vi "run.vi"(8 "error in (no error)":errorcluster, 11 "DL090503StimulatorScaffold in":refnum<class "StimulatorDL090503Scaffold.lvclass">) -> (0 "error out":errorcluster, 3 "DL090503StimulatorScaffold out":refnum<class "StimulatorDL090503Scaffold.lvclass">)   [LabVIEW 2010, in "StimulatorDL090503Scaffold.lvclass"]
uses:
  StimulatorDL090503Scaffold.lvclass
  schedule_entry_cluster.ctl
  common/classes/GenericToplevelComponent/GenericToplevelComponent/common_trigger_enum.ctl
  internal_trigger_enum.ctl
  StimulatorDL090503Scaffold.lvclass/StimulatorDL090503Scaffold.ctl
  GenericStimulator/GenericStimulator/GenericStimulator.lvclass
  common/classes/GenericComponent/GenericComponent/class_data.vi
  common/classes/GenericToplevelComponent/GenericToplevelComponent/GenericToplevelComponent.lvclass
  common/classes/GenericComponent/GenericComponent/GenericComponent.lvclass
panel:
  out "last statechart trigger":T1
  out "event loop time-out":i32
  in  "scheduled triggers":T2[](array[typedef])
  out "trigger schedule loop counter":i32
  out "statemachine  error":errorcluster
  out "statechart loop counter":i32
  out "finished?":bool
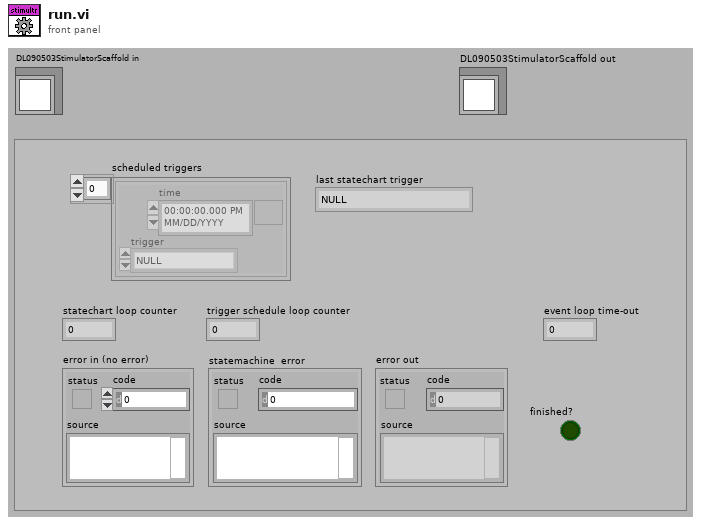
[diagram p1: front panel]
types:
  T1 = typedef "StimulatorDL090503Scaffold.lvclass/internal_trigger_enum.ctl" = enum16{"NULL", "initialise", "terminate", "start sweep", "stop sweep", "start stimulation", "stop stimulation"}
  T2 = typedef "StimulatorDL090503Scaffold.lvclass/schedule_entry_cluster.ctl" = cluster{"time":timestamp, "trigger":T3}
  T3 = typedef "GenericToplevelComponent.lvclass/common_trigger_enum.ctl" = enum16{"NULL", "initialise", "terminate", "fetch command", "fetch data", "attach observer", "register as observer", "detach observer", "acknowledge", "start", "stop", "sweep started", "sweep finished", "experiment started", "experiment stopped"}
  T4 = typedef "main_trigger_enum.ctl" = enum16{"NULL", "initialise", "terminate", "start", "stop", "change objective", "change experimentController", "change imagingMode", "save notebook", "started saving", "finished saving", "expCtr ready", "expCtr missing", "imgMd ready", "imgMd missing", "scanHd ready", "scanHd missing", "DAQ ready", "DAQ missing", "imgAsm ready", "imgAsm missing", "dataColl ready", "dataColl missing", "display ready", "display missing", "analysr ready", "analysr missing", "instrmnt ready", "instrmnt missing", "stimltr ready", "stimltr missing", "stage ready", "stage missing"}
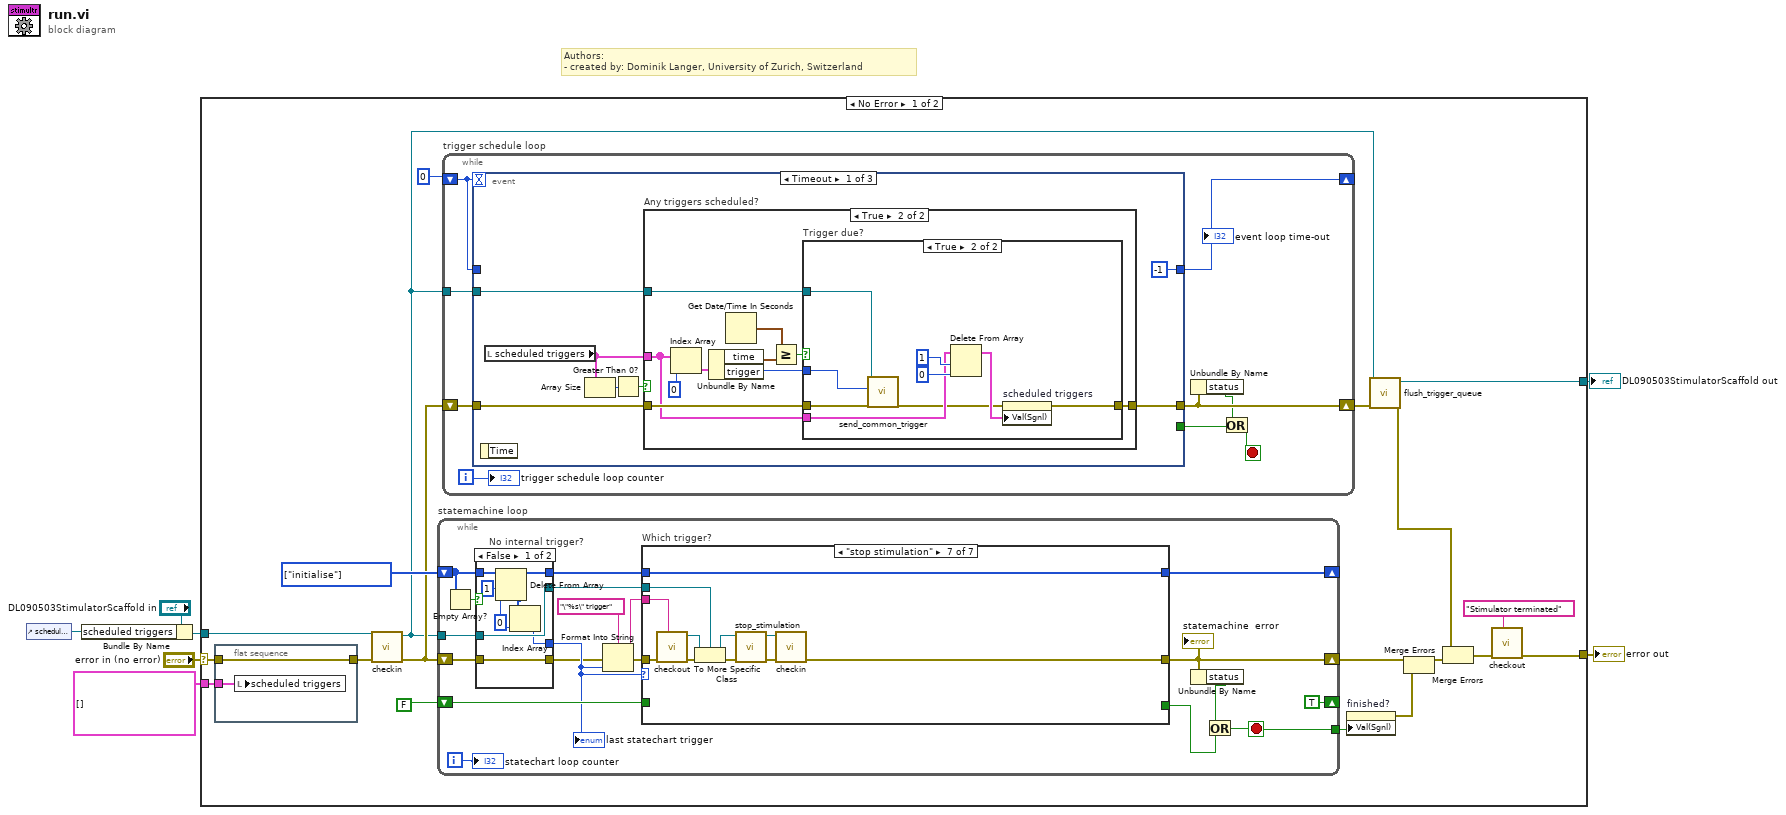
[diagram p0: block diagram]
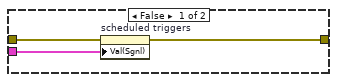
[diagram p3: hidden frame]
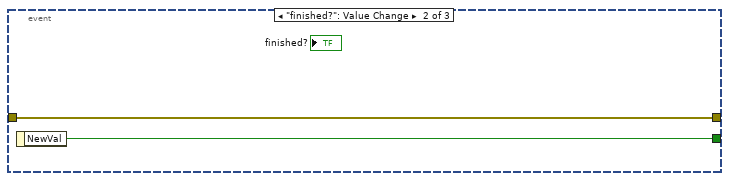
[diagram p4: hidden frame]
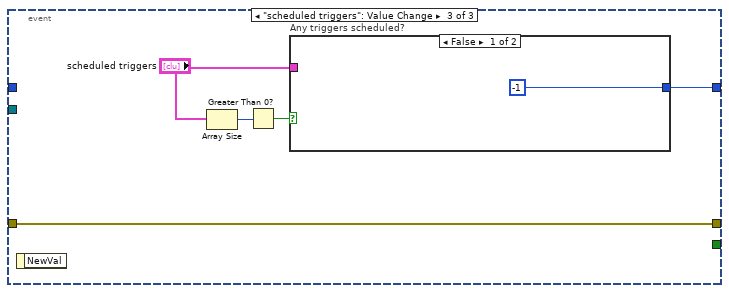
[diagram p5: hidden frame]
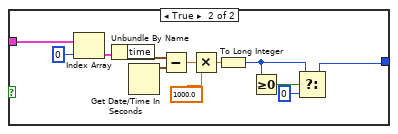
[diagram p6: hidden frame]
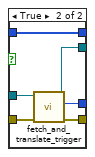
[diagram p7: hidden frame]
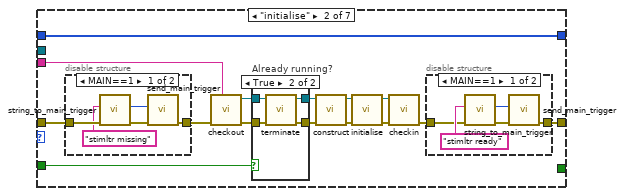
[diagram p9: hidden frame]
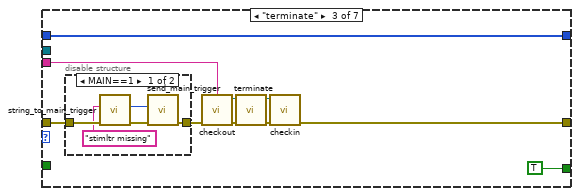
[diagram p13: hidden frame]
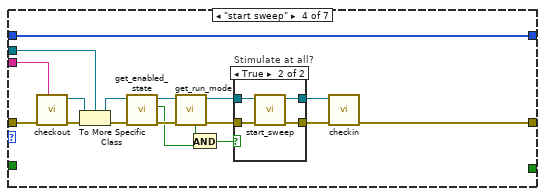
[diagram p15: hidden frame]
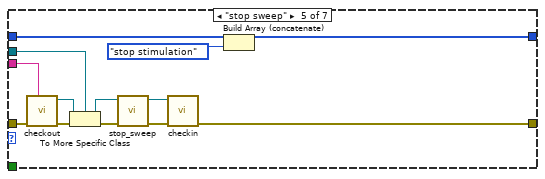
[diagram p17: hidden frame]
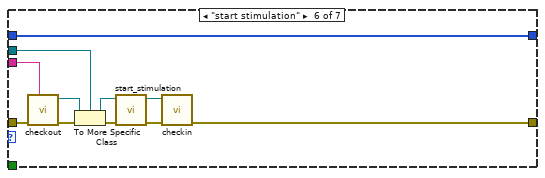
[diagram p18: hidden frame]
diagram:
  # "Authors: \n- created by: Dominik Langer, University of Zurich, Switzerland"
  n1 = control-ref of="scheduled triggers"() -> (w1:refnum<vi>)
  n2 = Bundle By Name(cluster="DL090503StimulatorScaffold in", "scheduled triggers"=w1) -> (w3:refnum<class "StimulatorDL090503Scaffold.lvclass">)
  n3 = case shown="No Error" "error in (no error)" {
    selector: "error in (no error)" -> [w23 w232]
    tunnel: [w15 w232] -> w6
    tunnel: w3 -> [w18 w231]
    tunnel: [w20 w231] -> w5
    tunnel: T2[] [] ("scheduled triggers") -> [w24 _]
    frame No Error {
      w10 = T1[] [enum."initialise"] items=["NULL", "initialise", "terminate", "start sweep", "stop sweep", "start stimulation", "stop stimulation"]
      n4 = flat-sequence {
        tunnel: w24 -> [w28]
        tunnel: w23 -> [w27]
        tunnel: [w27] -> w19
        frame #0 {
          n5 = local write "scheduled triggers"(w28) -> ()
        }
      }
      n6 = call-dynamic "checkin.vi"("error in (no error)"=w19, "GenericStimulator in"=w18) -> ("error out"=w9:errorcluster, "GenericStimulator out"=w8:refnum<class "StimulatorDL090503Scaffold.lvclass">)  [unwired: 8 in]
      n7 = while "statemachine loop" {
        shift-right: [TRUE] -> _
        shift-left: FALSE -> [w101]
        shift-right: [w100] -> w13
        shift-left: w9 -> [w104]
        tunnel: w8 -> [w103]
        tunnel: [w102] -> w17
        shift-right: [w91] -> _
        shift-left: w10 -> [w90]
        i -> [w105]
        stop <- w102 stop-if-true
        n8 = Empty Array?(array=w90) -> (empty?=w89:bool)
        n9 = case "No internal trigger?" shown="False" w89 {
          tunnel: w104 -> [w114 w120]
          tunnel: w103 -> [w113 w119]
          tunnel: [w109 w118] -> w97
          tunnel: [w114 w117] -> w96
          tunnel: [w113 w116] -> w92
          tunnel: w90 -> [w112 w115]
          tunnel: [w111 w115] -> w88
          frame False {
            w108 = 0 ("index")
            n10 = Delete From Array(array=w112, length=1, index=w108) -> (deleted portion=w110:T1[], array with subset deleted=w111:T1[])
            n11 = Index Array(array=w110, index=w108) -> (element=w109:T1)
          }
          frame True {
            n12 = call-dynamic "fetch_and_translate_trigger.vi"("error in (no error)"=w120, "StimulatorDL090503Scaffold in"=w119) -> ("error out"=w117:errorcluster, "statechart trigger"=w118:T1, "StimulatorDL090503Scaffold out"=w116:refnum<class "StimulatorDL090503Scaffold.lvclass">)  [unwired: 6 in, 1 out]
          }
        }
        "last statechart trigger" <- w97
        n13 = Format Into String(format string="\"%s\" trigger", error in=w96, w97) -> (resulting string=w93:string, error out=w95:errorcluster)  [unwired: 1 in]
        n14 = case "Which trigger?" shown="\"stop stimulation\"" w97 {
          tunnel: w95 -> [w122 w125 w157 w184 w200 w210 w223]
          tunnel: w101 -> [_ w128 _ _ _ _ _]
          tunnel: [w122 w126 w159 w183 w199 w209 w220] -> w100
          tunnel: [_ _ TRUE _ _ _ _] -> w99
          tunnel: w93 -> [_ w129 w160 w185 w202 w211 w221]
          tunnel: w92 -> [_ _ _ w182 w201 w212 w222]
          tunnel: w88 -> [w121 w123 w158 w181 w197 w219 w230]
          tunnel: [w121 w123 w158 w181 w196 w219 w230] -> w91
          frame "NULL", Default {
          }
          frame "initialise" {
            n15 = disable-structure shown="MAIN==1" {
              disable-tunnel: w125 -> [w141 w143]
              disable-tunnel: [w142 w143] -> w124
              frame condition #0 (active) {
                n16 = call "string_to_main_trigger.vi"("error in (no error)"=w141, "trigger string"="stimltr missing") -> ("error out"=w140:errorcluster, "main trigger"=w139:T4)  [unwired: 8 in]
                n17 = call "send_main_trigger.vi"("error in (no error)"=w140, "trigger"=w139) -> ("error out"=w142:errorcluster)  [unwired: 9 in]
              }
              frame condition #1 {
              }
            }
            n18 = call "checkout.vi"("locked by?"=w129, "error in (no error)"=w124) -> ("error out"=w134:errorcluster, "GenericStimulator out"=w136:refnum<class "GenericStimulator.lvclass">)  [unwired: 8 out]
            n19 = case "Already running?" shown="True" w128 {
              tunnel: w134 -> [w151 w155]
              tunnel: [w151 w154] -> w135
              tunnel: w136 -> [w150 w153]
              tunnel: [w150 w152] -> w137
              frame False {
              }
              frame True {
                n20 = call-dynamic "terminate.vi"("error in (no error)"=w155, "GenericPlugin in"=w153) -> ("error out"=w154:errorcluster, "GenericPlugin out"=w152:refnum<class "GenericStimulator.lvclass">)  [unwired: 8 out]
              }
            }
            n21 = call-dynamic "construct.vi"("error in (no error)"=w135, "GenericPlugin in"=w137) -> ("error out"=w132:errorcluster, "GenericPlugin out"=w133:refnum<class "GenericStimulator.lvclass">)  [unwired: 2 in, 6 out]
            n22 = call-dynamic "initialise.vi"("error in (no error)"=w132, "GenericPlugin in"=w133) -> ("error out"=w131:errorcluster, "GenericPlugin out"=w130:refnum<class "GenericStimulator.lvclass">)  [unwired: 8 out]
            n23 = call-dynamic "checkin.vi"("error in (no error)"=w131, "GenericStimulator in"=w130) -> ("error out"=w127:errorcluster)  [unwired: 8 in, 1 out]
            n24 = disable-structure shown="MAIN==1" {
              disable-tunnel: w127 -> [w145 w149]
              disable-tunnel: [w148 w149] -> w126
              frame condition #0 (active) {
                n25 = call "string_to_main_trigger.vi"("error in (no error)"=w145, "trigger string"="stimltr ready") -> ("error out"=w144:errorcluster, "main trigger"=w147:T4)  [unwired: 8 in]
                n26 = call "send_main_trigger.vi"("error in (no error)"=w144, "trigger"=w147) -> ("error out"=w148:errorcluster)  [unwired: 9 in]
              }
              frame condition #1 {
              }
            }
          }
          frame "terminate" {
            n27 = disable-structure shown="MAIN==1" {
              disable-tunnel: w157 -> [w169 w171]
              disable-tunnel: [w170 w171] -> w156
              frame condition #0 (active) {
                n28 = call "string_to_main_trigger.vi"("error in (no error)"=w169, "trigger string"="stimltr missing") -> ("error out"=w168:errorcluster, "main trigger"=w167:T4)  [unwired: 8 in]
                n29 = call "send_main_trigger.vi"("error in (no error)"=w168, "trigger"=w167) -> ("error out"=w170:errorcluster)  [unwired: 9 in]
              }
              frame condition #1 {
              }
            }
            n30 = call "checkout.vi"("locked by?"=w160, "error in (no error)"=w156) -> ("error out"=w164:errorcluster, "GenericStimulator out"=w163:refnum<class "GenericStimulator.lvclass">)  [unwired: 8 out]
            n31 = call-dynamic "terminate.vi"("error in (no error)"=w164, "GenericPlugin in"=w163) -> ("error out"=w161:errorcluster, "GenericPlugin out"=w162:refnum<class "GenericStimulator.lvclass">)  [unwired: 8 out]
            n32 = call-dynamic "checkin.vi"("error in (no error)"=w161, "GenericStimulator in"=w162) -> ("error out"=w159:errorcluster)  [unwired: 8 in, 1 out]
          }
          frame "start sweep" {
            n33 = call "checkout.vi"("locked by?"=w185, "error in (no error)"=w184) -> ("error out"=w187:errorcluster, "GenericStimulator out"=w186:refnum<class "GenericStimulator.lvclass">)  [unwired: 8 out]
            n34 = To More Specific Class(target class=w182, reference=w186, error in=w187) -> (specific class reference=w174:refnum<class "StimulatorDL090503Scaffold.lvclass">, error out=w177:errorcluster)
            n35 = call-dynamic "get_enabled_state.vi"("error in (no error)"=w177, "GenericStimulator in"=w174) -> ("error out"=w180:errorcluster, "stimulator enabled?"=w179:bool, "GenericStimulator out"=w175:refnum<class "StimulatorDL090503Scaffold.lvclass">)  [unwired: 7 in]
            n36 = call "get_run_mode.vi"("error in (no error)"=w180, "GenericPlugin in"=w175) -> ("error out"=w176:errorcluster, "GenericPlugin out"=w173:refnum<class "StimulatorDL090503Scaffold.lvclass">, "is NOT free run?"=w178:bool)  [unwired: 5 in, 2 out]
            n37 = And(x=w178, y=w179) -> (x .and. y?=w172:bool)
            n38 = case "Stimulate at all?" shown="True" w172 {
              tunnel: [w190 w195] -> w189
              tunnel: [w191 w194] -> w188
              tunnel: w176 -> [w190 w193]
              tunnel: w173 -> [w191 w192]
              frame False {
              }
              frame True {
                n39 = call-dynamic "start_sweep.vi"("error in (no error)"=w193, "DL090503StimulatorScaffold in"=w192) -> ("error out"=w195:errorcluster, "DL090503StimulatorScaffold out"=w194:refnum<class "StimulatorDL090503Scaffold.lvclass">)  [unwired: 8 out]
              }
            }
            n40 = call-dynamic "checkin.vi"("error in (no error)"=w189, "GenericStimulator in"=w188) -> ("error out"=w183:errorcluster)  [unwired: 8 in, 1 out]
          }
          frame "stop sweep" {
            n41 = call "checkout.vi"("locked by?"=w202, "error in (no error)"=w200) -> ("error out"=w206:errorcluster, "GenericStimulator out"=w205:refnum<class "GenericStimulator.lvclass">)  [unwired: 8 out]
            n42 = To More Specific Class(target class=w201, reference=w205, error in=w206) -> (specific class reference=w204:refnum<class "StimulatorDL090503Scaffold.lvclass">, error out=w203:errorcluster)
            n43 = call-dynamic "stop_sweep.vi"("error in (no error)"=w203, "DL090503StimulatorScaffold in"=w204) -> ("error out"=w208:errorcluster, "DL090503StimulatorScaffold out"=w207:refnum<class "StimulatorDL090503Scaffold.lvclass">)  [unwired: 8 out]
            n44 = call-dynamic "checkin.vi"("error in (no error)"=w208, "GenericStimulator in"=w207) -> ("error out"=w199:errorcluster)  [unwired: 8 in, 1 out]
            n45 = Build Array (concatenate)(w197, internal_trigger_enum."stop stimulation" ("trigger")) -> (w196:T1[])
          }
          frame "start stimulation" {
            n46 = call "checkout.vi"("locked by?"=w211, "error in (no error)"=w210) -> ("error out"=w218:errorcluster, "GenericStimulator out"=w217:refnum<class "GenericStimulator.lvclass">)  [unwired: 8 out]
            n47 = To More Specific Class(target class=w212, reference=w217, error in=w218) -> (specific class reference=w215:refnum<class "StimulatorDL090503Scaffold.lvclass">, error out=w216:errorcluster)
            n48 = call-dynamic "start_stimulation.vi"("error in (no error)"=w216, "DL090503StimulatorScaffold in"=w215) -> ("error out"=w214:errorcluster, "DL090503StimulatorScaffold out"=w213:refnum<class "StimulatorDL090503Scaffold.lvclass">)  [unwired: 8 out]
            n49 = call-dynamic "checkin.vi"("error in (no error)"=w214, "GenericStimulator in"=w213) -> ("error out"=w209:errorcluster)  [unwired: 8 in, 1 out]
          }
          frame "stop stimulation" {
            n50 = call "checkout.vi"("locked by?"=w221, "error in (no error)"=w223) -> ("error out"=w229:errorcluster, "GenericStimulator out"=w228:refnum<class "GenericStimulator.lvclass">)  [unwired: 8 out]
            n51 = To More Specific Class(target class=w222, reference=w228, error in=w229) -> (specific class reference=w226:refnum<class "StimulatorDL090503Scaffold.lvclass">, error out=w227:errorcluster)
            n52 = call-dynamic "stop_stimulation.vi"("error in (no error)"=w227, "DL090503StimulatorScaffold in"=w226) -> ("error out"=w225:errorcluster, "DL090503StimulatorScaffold out"=w224:refnum<class "StimulatorDL090503Scaffold.lvclass">)  [unwired: 8 out]
            n53 = call-dynamic "checkin.vi"("error in (no error)"=w225, "GenericStimulator in"=w224) -> ("error out"=w220:errorcluster)  [unwired: 8 in, 1 out]
          }
        }
        "statemachine  error" <- w100
        n54 = Unbundle By Name(w100) -> ("status"=w98:bool)
        n55 = Or(x=w98, y=w99) -> (x .or. y?=w102:bool)
        "statechart loop counter" <- w105
      }
      n56 = while "trigger schedule loop" {
        tunnel: w8 -> [w29]
        shift-right: [w35] -> _
        shift-left: 0 -> [w37]
        shift-right: [w33] -> w21
        shift-left: w9 -> [w36]
        i -> [w34]
        stop <- w30 stop-if-true
        n57 = event shown="[0] Timeout" {
          selector: _ -> [_ _ _]
          dyn-events: _ -> [_ _ _]
          timeout: w37 -> [_ _ _]
          tunnel: w37 -> [_ _ _]
          tunnel: w36 -> [w42 w69 w74]
          tunnel: [w41 w69 w74] -> w33
          tunnel: [-1 _ w73] -> w35
          tunnel: [_ w68 _] -> w31
          tunnel: w29 -> [w38 _ _]
          event Timeout {
            n58 = event-data() -> ()  [unwired: 2 out]
            n59 = local read "scheduled triggers"() -> (w44:T2[])
            n60 = Array Size(array=w44) -> (size(s)=w43:i32)
            n61 = Greater Than 0?(x=w43) -> (x > 0?=w40:bool)
            n62 = case "Any triggers scheduled?" shown="True" w40 {
              tunnel: w44 -> [_ w47]
              tunnel: w42 -> [w45 w54]
              tunnel: [w45 w53] -> w41
              tunnel: w38 -> [_ w46]
              frame False {
              }
              frame True {
                n63 = Index Array(array=w47, index=0) -> (element=w51:T2)
                n64 = Unbundle By Name(w51) -> ("time"=w49:timestamp, "trigger"=w52:T3)
                n65 = Get Date/Time In Seconds() -> (seconds since 1Jan1904=w50:timestamp)
                n66 = Greater Or Equal?(x=w50, y=w49) -> (x >= y?=w48:bool)
                n67 = case "Trigger due?" shown="True" w48 {
                  tunnel: w54 -> [w57 w62]
                  tunnel: [w56 w64] -> w53
                  tunnel: w52 -> [_ w60]
                  tunnel: w47 -> [w58 w65]
                  tunnel: w46 -> [_ w59]
                  frame False {
                    n68 = property on="scheduled triggers" class="Arr (strict)"(error in=w57, "Val(Sgnl)"=w58) -> (error out=w56:errorcluster)  [unwired: 1 in, 1 out]
                  }
                  frame True {
                    n69 = call-dynamic "send_common_trigger.vi"("error in (no error)"=w62, "trigger"=w60, "GenericToplevelComponent in"=w59) -> ("error out"=w61:errorcluster)  [unwired: 6 in, 2 out]
                    n70 = Delete From Array(array=w65, length=1, index=0) -> (array with subset deleted=w63:T2[])  [unwired: 1 out]
                    n71 = property on="scheduled triggers" class="Arr (strict)"(error in=w61, "Val(Sgnl)"=w63) -> (error out=w64:errorcluster)  [unwired: 1 in, 1 out]
                  }
                }
              }
            }
          }
          event "finished?": Value Change {
            n72 = event-data() -> ("NewVal"=w68:bool)  [unwired: 1 out]
          }
          event "scheduled triggers": Value Change {
            n73 = event-data() -> ()  [unwired: 2 out]
            n74 = Array Size(array="scheduled triggers") -> (size(s)=w71:i32)
            n75 = Greater Than 0?(x=w71) -> (x > 0?=w70:bool)
            n76 = case "Any triggers scheduled?" shown="False" w70 {
              tunnel: [-1 w78] -> w73
              tunnel: "scheduled triggers" -> [_ w83]
              frame False {
              }
              frame True {
                n77 = Index Array(array=w83, index=0) -> (element=w86:T2)
                n78 = Unbundle By Name(w86) -> ("time"=w85:timestamp)
                n79 = Get Date/Time In Seconds() -> (seconds since 1Jan1904=w84:timestamp)
                n80 = Subtract(x=w85, y=w84) -> (x-y=w82:dbl)
                n81 = Multiply(x=w82, y=1000.0) -> (x*y=w81:dbl)
                n82 = To Long Integer(number=w81) -> (32bit integer=w77:i32)
                n83 = Greater Or Equal To 0?(x=w77) -> (x >= 0?=w79:bool)
                n84 = Select(t=w77, s=w79, f=0) -> (s? t:f=w78:i32)
              }
            }
          }
        }
        "event loop time-out" <- w35
        n85 = Unbundle By Name(w33) -> ("status"=w32:bool)
        n86 = Or(x=w32, y=w31) -> (x .or. y?=w30:bool)
        "trigger schedule loop counter" <- w34
      }
      n87 = property on="finished?" class="Bool (strict)"("Val(Sgnl)"=w17) -> (error out=w12:errorcluster)  [unwired: 2 in, 1 out]
      n88 = call-dynamic "flush_trigger_queue.vi"("error in (no error)"=w21, "GenericToplevelComponent in"=w8) -> ("error out"=w22:errorcluster, "GenericToplevelComponent out"=w20:refnum<class "StimulatorDL090503Scaffold.lvclass">)  [unwired: 8 in]
      n89 = Merge Errors(w13, w12) -> (w11:errorcluster)
      n90 = Merge Errors(w22, w11) -> (w16:errorcluster)
      n91 = call "checkout.vi"("locked by?"="Stimulator terminated", "error in (no error)"=w16) -> ("error out"=w15:errorcluster)  [unwired: 9 out]
    }
    frame Error {
    }
  }
  "error out" <- w6
  "DL090503StimulatorScaffold out" <- w5
